vi "气象全局变量.vi"() -> ()   [LabVIEW 2016, in "AIRMAR WeatherCaster.lvlib"]
uses:
  AIRMAR WeatherCaster.lvlib
panel:
  in  "环境变量":cluster{"电压":dbl, "室温":dbl, "湿度":dbl}={"电压"=12.0, "室温"=25.0, "湿度"=75.0}
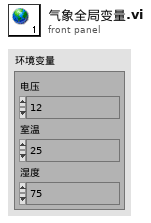
[diagram p1: front panel]
diagram:
